vi "Write Log Data.vi"(8 "error in":errorcluster, 10 "Log Data":T1, 11 "TDMS in":refnum<class "TDMS.lvclass">) -> (0 "error out":errorcluster, 3 "TDMS out":refnum<class "TDMS.lvclass">)   [LabVIEW 2017, in "Report_lib.lvlib" / "TDMS.lvclass"]
uses:
  TDMS.lvclass
  TDMS.lvclass/TDMS.ctl
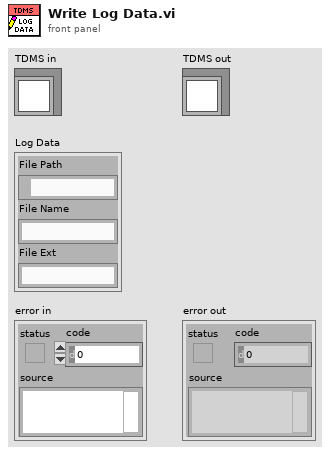
[diagram p1: front panel]
types:
  T1 = cluster{"File Path":path, "File Name":string, "File Ext":string}
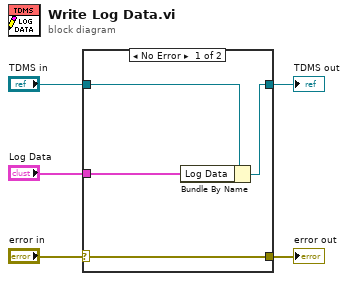
[diagram p0: block diagram]
diagram:
  n1 = case shown="No Error" "error in" {
    selector: "error in" -> [w9 w10]
    tunnel: [w9 w10] -> w4
    tunnel: [w7 w11] -> w2
    tunnel: "TDMS in" -> [w8 w11]
    tunnel: "Log Data" -> [w6 _]
    frame No Error {
      n2 = Bundle By Name(cluster=w8, "Log Data"=w6) -> (w7:refnum<class "TDMS.lvclass">)
    }
    frame Error {
    }
  }
  "error out" <- w4
  "TDMS out" <- w2
